vi "Edit CDMA2000 FW Channel Setup.vi"(0 "VISA Resource Name":refnum<visa-resource-name>, 1 "Insert (1: Append)":enum16{"Init", "Append", "Channel Number"}(ring)=enum."Append", 2 "Channel Number (1)":i32=1, 3 "Channel Type (1: Pilot)":T1(ring)=enum."Pilot", 4 "Config (3)":i32=3, 5 "error in (no error)":errorcluster {"code" format="%.0x"}, 6 "Data Rate (38400)":i32=38400, 7 "PN Offset  (0)":dbl, 8 "Walsh  (0)":i32, 9 "Data Type (0: Random)":enum16{"Random", "User"}(ring), 10 "Power  (-7.0)":dbl=-7.0, 11 "Data Value  (0000000)":i32 format="%b") -> (14 "VISA Resource Name Out":refnum<visa-resource-name>, 19 "error out":errorcluster {"code" format="%.0x"})   [LabVIEW 2012, in "Agilent ESG Series.lvlib"]
doc: "This VI is used to configure the forward channel parameters.\n\nThis VI is valid only on instruments E44xxB with the 101 option or on instrument E4438C with option 401."
uses:
  <instrlib>/Agilent ESG Series/Agilent ESG Series.lvlib
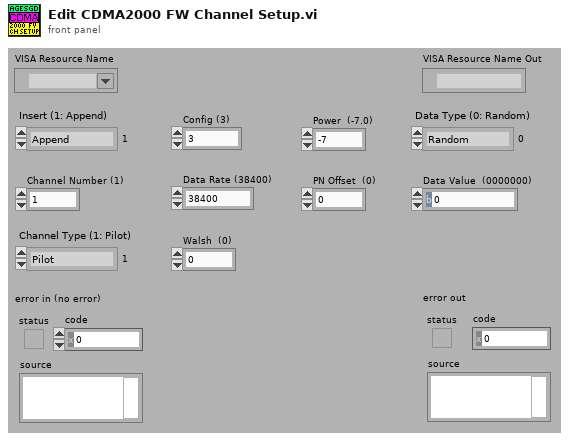
[diagram p1: front panel]
types:
  T1 = enum16{"Paging", "Pilot", "Sync", "Traffic", "S1 Traffic", "S2 Traffic"}
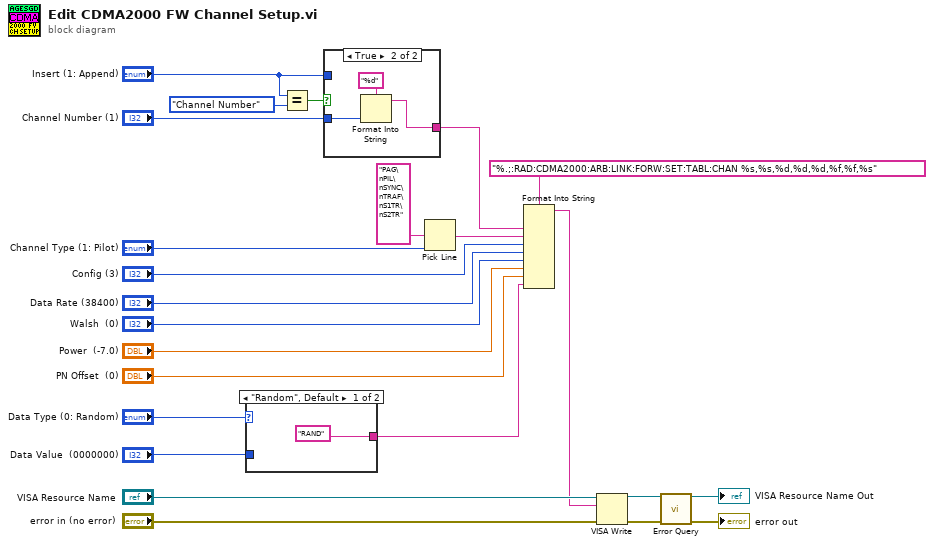
[diagram p0: block diagram]
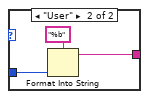
[diagram p2: hidden frame]
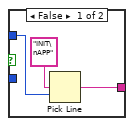
[diagram p3: hidden frame]
diagram:
  n1 = case shown="\"Random\", Default" "Data Type (0: Random)" {
    tunnel: ["RAND" ("multi-line string") w27] -> w7
    tunnel: "Data Value  (0000000)" -> [_ w26]
    frame "Random", Default {
    }
    frame "User" {
      n2 = Format Into String(format string="%b", w26) -> (resulting string=w27:string)  [unwired: 2 in, 1 out]
    }
  }
  n3 = Equal?(x="Insert (1: Append)", y=enum16{"Init", "Append", "Channel Number"}."Channel Number" ("Insert (1: Append)")) -> (x = y?=w21:bool)
  n4 = case shown="True" w21 {
    tunnel: "Channel Number (1)" -> [_ w34]
    tunnel: [w29 w32] -> w18
    tunnel: "Insert (1: Append)" -> [w30 _]
    frame False {
      n5 = Pick Line(multi-line string="INIT\nAPP", line index=w30) -> (output string=w29:string)  [unwired: 1 in]
    }
    frame True {
      n6 = Format Into String(format string="%d", w34) -> (resulting string=w32:string)  [unwired: 2 in, 1 out]
    }
  }
  n7 = Pick Line(multi-line string="PAG\nPIL\nSYNC\nTRAF\nS1TR\nS2TR", line index="Channel Type (1: Pilot)") -> (output string=w15:string)  [unwired: 1 in]
  n8 = Format Into String(format string="%.;:RAD:CDMA2000:ARB:LINK:FORW:SET:TABL:CHAN %s,%s,%d,%d,%d,%f,%f,%s", w18, w15, "Config (3)", "Data Rate (38400)", "Walsh  (0)", "Power  (-7.0)", "PN Offset  (0)", w7) -> (resulting string=w5:string)  [unwired: 2 in, 1 out]
  n9 = VISA Write(VISA resource name="VISA Resource Name", write buffer=w5, error in (no error)="error in (no error)") -> (VISA resource name out=w4:refnum<visa-resource-name>, error out=w1:errorcluster)  [unwired: 1 out]
  n10 = call <instrlib>:"Error Query.vi"("VISA Resource Name"=w4, "error in (no error)"=w1) -> ("VISA Resource Name Out"=→"VISA Resource Name Out":refnum<visa-resource-name>, "error out"=→"error out":errorcluster)  [unwired: 10 in, 2 out]
